vi "例4-11.vi"() -> ()   [LabVIEW 2019]
panel:
  out "输出字符串":string
  in  "输入字符串":string="conversion STR"
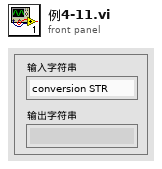
[diagram p1: front panel]
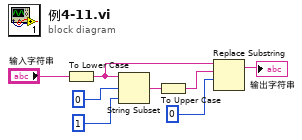
[diagram p0: block diagram]
diagram:
  n1 = To Lower Case(string="输入字符串") -> (all lower case string=w4:string)
  n2 = String Subset(string=w4, offset (0)=0, length (rest)=1) -> (substring=w7:string)
  n3 = To Upper Case(1:w7) -> (0:w3:string)
  n4 = Replace Substring(3:0, 4:w3, 5:w4) -> (1:→"输出字符串":string)  [unwired: 1 in, 1 out]
